vi "CAD@SetRobotBase__Parameter.vi"(1 "ParamterIn":string) -> (0 "ParamterOut":string)   [LabVIEW 2019]
panel:
  in  "Position":string(combo)
  in  "RobotName":string(combo)
  in  "Confirm":bool
  # "CAD@SetRobotBase $Robot,$PointName\nCAD@SetRobotBase $Robot,(X,Y,Z,U,V,W)"
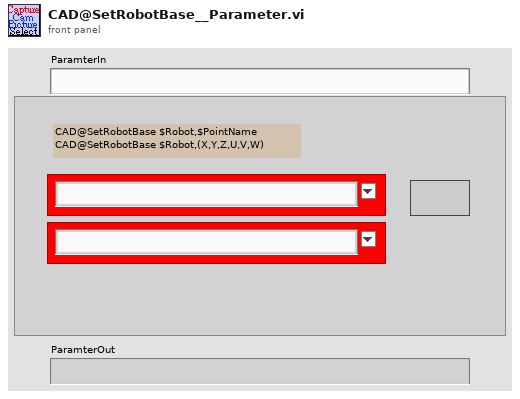
[diagram p1: front panel]
types:
  T1 = enum16{"Get", "UpdatePointS", "Init", "UpdateIndex", "GetCurrent&Index+1", "GetWithIndex", "ChkLast", "GetCurrent"}
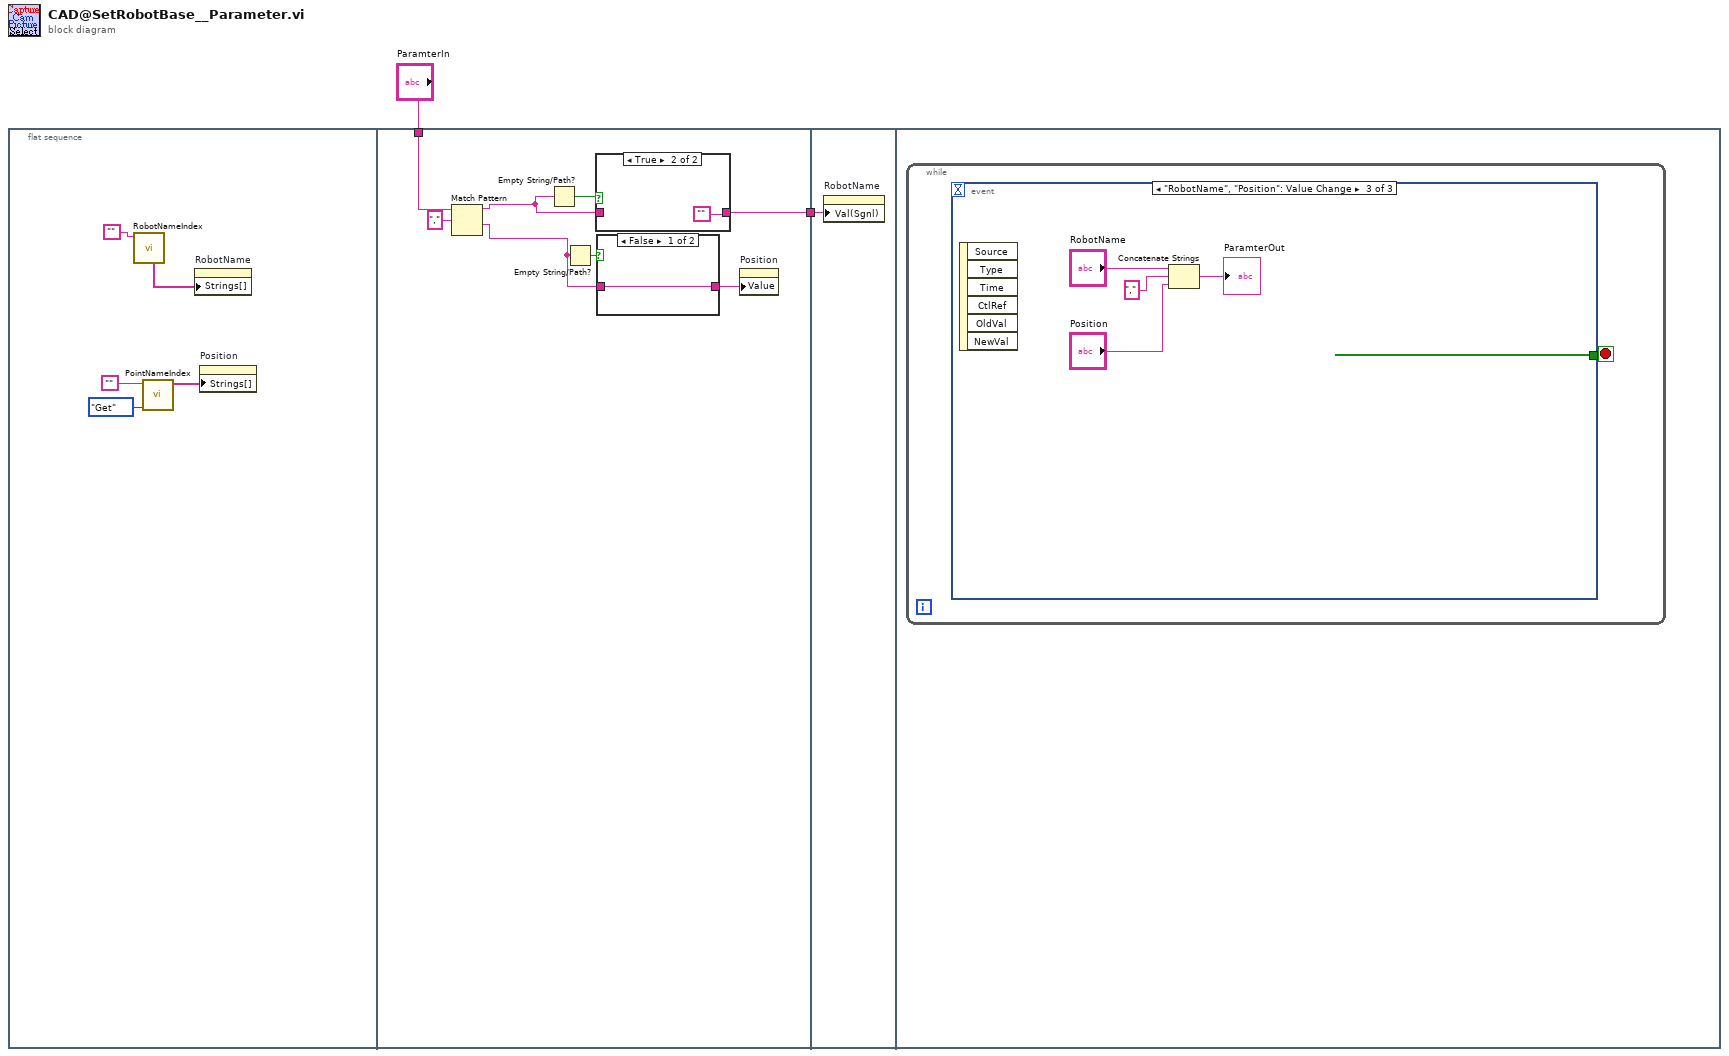
[diagram p0: block diagram]
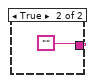
[diagram p2: hidden frame]
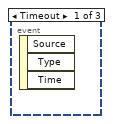
[diagram p4: hidden frame]
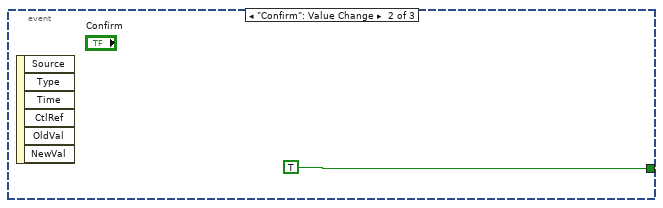
[diagram p5: hidden frame]
diagram:
  n1 = flat-sequence {
    tunnel: "ParamterIn" -> [w11]
    tunnel: [w13] -> w1
    tunnel: w1 -> [w20]
    frame #0 {
      n2 = call "RobotNameIndex.vi"("RobotName"="") -> ("RobotNameList"=w6:string[])  [unwired: 8 in, 2 out]
      n3 = call "PointNameIndex.vi"("OP"=T1."Get", "PointName"="") -> ("PointNameList"=w4:string[])  [unwired: 4 in, 5 out]
      n4 = property on="RobotName" class="CmbBox"("Strings[]"=w6) -> ()  [unwired: 2 in, 2 out]
      n5 = property on="Position" class="CmbBox"("Strings[]"=w4) -> ()  [unwired: 2 in, 2 out]
    }
    frame #1 {
      n6 = Match Pattern(string=w11, regular expression=",") -> (before substring=w9:string, after substring=w8:string)  [unwired: 1 in, 2 out]
      n7 = Empty String/Path?(string/path=w9) -> (empty?=w15:bool)
      n8 = Empty String/Path?(string/path=w8) -> (empty?=w14:bool)
      n9 = case shown="True" w15 {
        tunnel: w9 -> [w18 _]
        tunnel: [w18 ""] -> w13
        frame False {
        }
        frame True {
        }
      }
      n10 = case shown="False" w14 {
        tunnel: [w16 ""] -> w12
        tunnel: w8 -> [w16 _]
        frame False {
        }
        frame True {
        }
      }
      n11 = property on="Position" class="CmbBox"("Value"=w12) -> ()  [unwired: 2 in, 2 out]
    }
    frame #2 {
      n12 = property on="RobotName" class="CmbBox"("Val(Sgnl)"=w20) -> ()  [unwired: 2 in, 2 out]
    }
    frame #3 {
      n13 = while {
        stop <- w21 stop-if-true
        n14 = event shown="[2] \"RobotName\", \"Position\": Value Change" {
          selector: _ -> [_ _ _]
          dyn-events: _ -> [_ _ _]
          timeout: _ -> [_ _ _]
          tunnel: [_ TRUE _] -> w21
          event Timeout {
            n15 = event-data() -> ()  [unwired: 1 in, 3 out]
          }
          event "Confirm": Value Change {
            n16 = event-data() -> ()  [unwired: 1 in, 6 out]
          }
          event "RobotName", "Position": Value Change {
            n17 = event-data() -> ()  [unwired: 1 in, 6 out]
            n18 = Concatenate Strings("RobotName", "," ("element"), "Position") -> (→"ParamterOut":string)
          }
        }
      }
    }
  }
